vi "Scan from Function.vi"(0 "initial string":string, 1 "Syntax Format":T1, 11 "error in":errorcluster) -> (4 "resulting string":string, 6 "Variables Name":string[](array[string]), 8 "Variables Value":string[](array[string]), 15 "error out":errorcluster)   [LabVIEW 2019]
uses:
  Scan Syntax Format.ctl
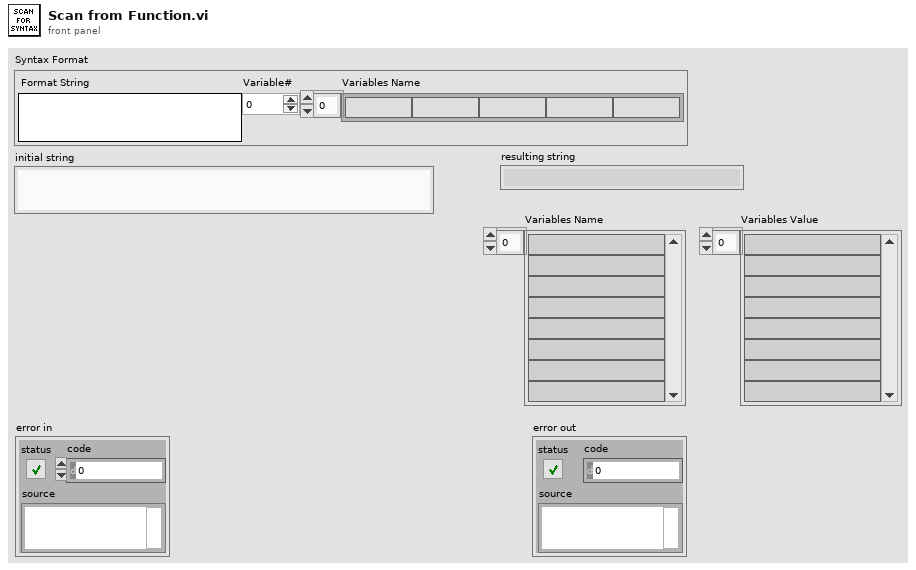
[diagram p1: front panel]
types:
  T1 = typedef "Scan Syntax Format.ctl" = cluster{"Format String":string, "Variable#":i32, "Variables Name":string[]}
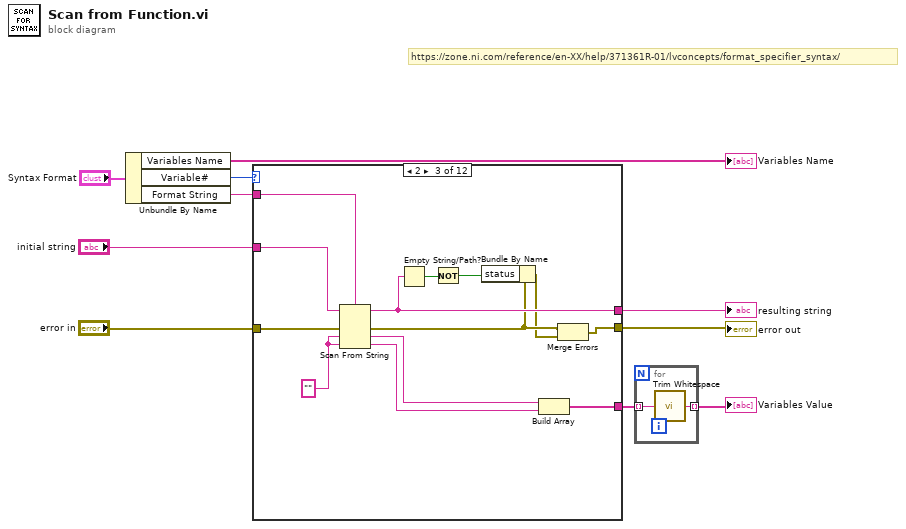
[diagram p0: block diagram]
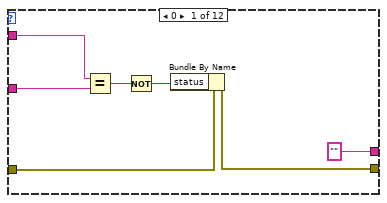
[diagram p2: hidden frame]
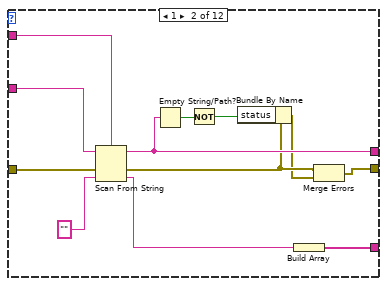
[diagram p3: hidden frame]
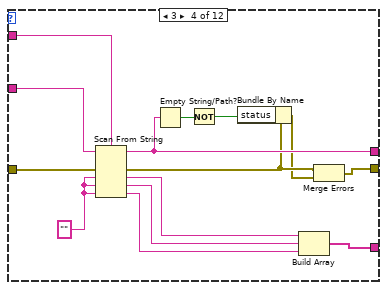
[diagram p4: hidden frame]
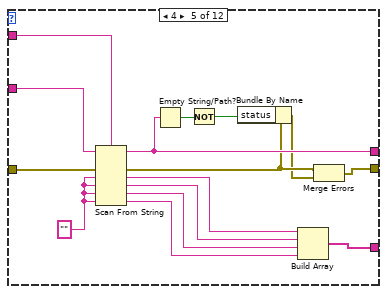
[diagram p5: hidden frame]
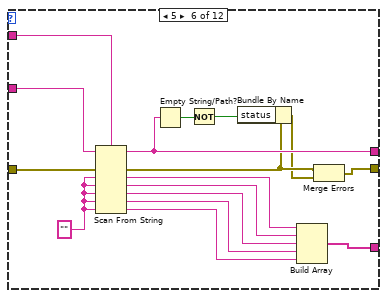
[diagram p6: hidden frame]
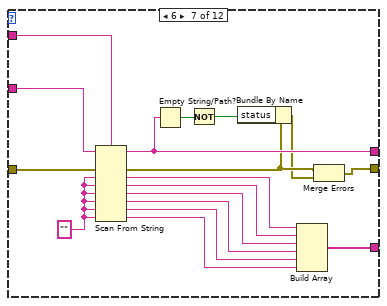
[diagram p7: hidden frame]
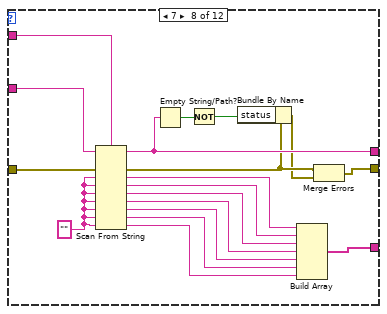
[diagram p8: hidden frame]
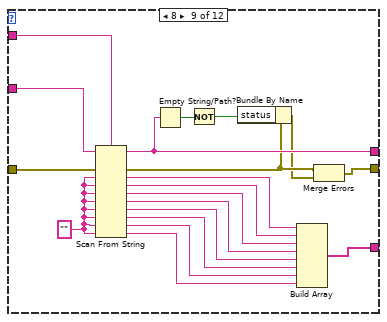
[diagram p9: hidden frame]
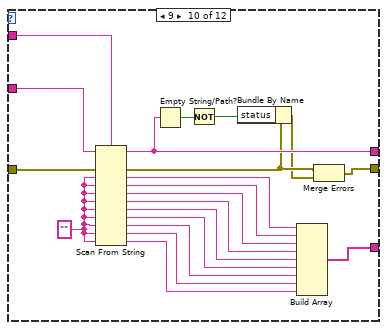
[diagram p10: hidden frame]
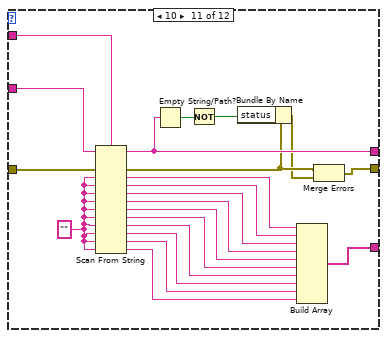
[diagram p11: hidden frame]
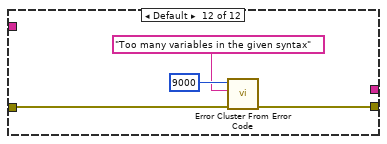
[diagram p12: hidden frame]
diagram:
  # "https://zone.ni.com/reference/en-XX/help/371361R-01/lvconcepts/format_specifier_syntax/"
  n1 = Unbundle By Name("Syntax Format") -> ("Variables Name"=→"Variables Name":string[], "Variable#"=w5:i32, "Format String"=w6:string)
  n2 = case shown="2" w5 {
    tunnel: "initial string" -> [w16 w29 w42 w56 w71 w87 w104 w122 w141 w161 w182 _]
    tunnel: "error in" -> [w14 w27 w41 w55 w70 w86 w103 w121 w140 w160 w181 w186]
    tunnel: ["" w26 w40 w54 w69 w85 w102 w120 w139 w159 w180 _] -> w8
    tunnel: [w13 w20 w34 w48 w63 w79 w96 w114 w133 w153 w174 w185] -> w1
    tunnel: w6 -> [w17 w23 w37 w51 w66 w82 w99 w117 w136 w156 w177 _]
    tunnel: [_ w18 w30 w43 w57 w72 w90 w108 w127 w147 w168 _] -> w3
    frame 0 {
      n3 = Equal?(x=w17, y=w16) -> (x = y?=w12:bool)
      n4 = Not(x=w12) -> (.not. x?=w11:bool)
      n5 = Bundle By Name(cluster=w14, "status"=w11) -> (w13:errorcluster)
    }
    frame 1 {
      n6 = Scan From String(format string=w23, input string=w29, error in=w27, default 1="") -> (remaining string=w26:string, error out=w22:errorcluster, output 1=w19:string)  [unwired: 1 in, 1 out]
      n7 = Empty String/Path?(string/path=w26) -> (empty?=w25:bool)
      n8 = Not(x=w25) -> (.not. x?=w24:bool)
      n9 = Bundle By Name(cluster=w22, "status"=w24) -> (w21:errorcluster)
      n10 = Build Array(w19) -> (w18:string[])
      n11 = Merge Errors(w22, w21) -> (w20:errorcluster)
    }
    frame 2 {
      w33 = ""
      n12 = Scan From String(format string=w37, input string=w42, error in=w41, default 1=w33, default 2=w33) -> (remaining string=w40:string, error out=w36:errorcluster, output 1=w32:string, output 2=w31:string)  [unwired: 1 in, 1 out]
      n13 = Empty String/Path?(string/path=w40) -> (empty?=w39:bool)
      n14 = Not(x=w39) -> (.not. x?=w38:bool)
      n15 = Bundle By Name(cluster=w36, "status"=w38) -> (w35:errorcluster)
      n16 = Build Array(w32, w31) -> (w30:string[])
      n17 = Merge Errors(w36, w35) -> (w34:errorcluster)
    }
    frame 3 {
      w47 = ""
      n18 = Scan From String(format string=w51, input string=w56, error in=w55, default 1=w47, default 2=w47, default 3=w47) -> (remaining string=w54:string, error out=w50:errorcluster, output 1=w46:string, output 2=w45:string, output 3=w44:string)  [unwired: 1 in, 1 out]
      n19 = Empty String/Path?(string/path=w54) -> (empty?=w53:bool)
      n20 = Not(x=w53) -> (.not. x?=w52:bool)
      n21 = Bundle By Name(cluster=w50, "status"=w52) -> (w49:errorcluster)
      n22 = Build Array(w46, w45, w44) -> (w43:string[])
      n23 = Merge Errors(w50, w49) -> (w48:errorcluster)
    }
    frame 4 {
      w62 = ""
      n24 = Scan From String(format string=w66, input string=w71, error in=w70, default 1=w62, default 2=w62, default 3=w62, default 4=w62) -> (remaining string=w69:string, error out=w65:errorcluster, output 1=w61:string, output 2=w60:string, output 3=w59:string, output 4=w58:string)  [unwired: 1 in, 1 out]
      n25 = Empty String/Path?(string/path=w69) -> (empty?=w68:bool)
      n26 = Not(x=w68) -> (.not. x?=w67:bool)
      n27 = Bundle By Name(cluster=w65, "status"=w67) -> (w64:errorcluster)
      n28 = Build Array(w61, w60, w59, w58) -> (w57:string[])
      n29 = Merge Errors(w65, w64) -> (w63:errorcluster)
    }
    frame 5 {
      w78 = ""
      n30 = Scan From String(format string=w82, input string=w87, error in=w86, default 1=w78, default 2=w78, default 3=w78, default 4=w78, default 5=w78) -> (remaining string=w85:string, error out=w81:errorcluster, output 1=w77:string, output 2=w76:string, output 3=w75:string, output 4=w74:string, output 5=w73:string)  [unwired: 1 in, 1 out]
      n31 = Empty String/Path?(string/path=w85) -> (empty?=w84:bool)
      n32 = Not(x=w84) -> (.not. x?=w83:bool)
      n33 = Bundle By Name(cluster=w81, "status"=w83) -> (w80:errorcluster)
      n34 = Build Array(w77, w76, w75, w74, w73) -> (w72:string[])
      n35 = Merge Errors(w81, w80) -> (w79:errorcluster)
    }
    frame 6 {
      w89 = ""
      n36 = Scan From String(format string=w99, input string=w104, error in=w103, default 1=w89, default 2=w89, default 3=w89, default 4=w89, default 5=w89, default 6=w89) -> (remaining string=w102:string, error out=w98:errorcluster, output 1=w95:string, output 2=w94:string, output 3=w93:string, output 4=w92:string, output 5=w91:string, output 6=w88:string)  [unwired: 1 in, 1 out]
      n37 = Empty String/Path?(string/path=w102) -> (empty?=w101:bool)
      n38 = Not(x=w101) -> (.not. x?=w100:bool)
      n39 = Bundle By Name(cluster=w98, "status"=w100) -> (w97:errorcluster)
      n40 = Build Array(w95, w94, w93, w92, w91, w88) -> (w90:string[])
      n41 = Merge Errors(w98, w97) -> (w96:errorcluster)
    }
    frame 7 {
      w105 = ""
      n42 = Scan From String(format string=w117, input string=w122, error in=w121, default 1=w105, default 2=w105, default 3=w105, default 4=w105, default 5=w105, default 6=w105, default 7=w105) -> (remaining string=w120:string, error out=w116:errorcluster, output 1=w113:string, output 2=w112:string, output 3=w111:string, output 4=w110:string, output 5=w109:string, output 6=w107:string, output 7=w106:string)  [unwired: 1 in, 1 out]
      n43 = Empty String/Path?(string/path=w120) -> (empty?=w119:bool)
      n44 = Not(x=w119) -> (.not. x?=w118:bool)
      n45 = Bundle By Name(cluster=w116, "status"=w118) -> (w115:errorcluster)
      n46 = Build Array(w113, w112, w111, w110, w109, w107, w106) -> (w108:string[])
      n47 = Merge Errors(w116, w115) -> (w114:errorcluster)
    }
    frame 8 {
      w123 = ""
      n48 = Scan From String(format string=w136, input string=w141, error in=w140, default 1=w123, default 2=w123, default 3=w123, default 4=w123, default 5=w123, default 6=w123, default 7=w123, default 8=w123) -> (remaining string=w139:string, error out=w135:errorcluster, output 1=w132:string, output 2=w131:string, output 3=w130:string, output 4=w129:string, output 5=w128:string, output 6=w126:string, output 7=w125:string, output 8=w124:string)  [unwired: 1 in, 1 out]
      n49 = Empty String/Path?(string/path=w139) -> (empty?=w138:bool)
      n50 = Not(x=w138) -> (.not. x?=w137:bool)
      n51 = Bundle By Name(cluster=w135, "status"=w137) -> (w134:errorcluster)
      n52 = Build Array(w132, w131, w130, w129, w128, w126, w125, w124) -> (w127:string[])
      n53 = Merge Errors(w135, w134) -> (w133:errorcluster)
    }
    frame 9 {
      w142 = ""
      n54 = Scan From String(format string=w156, input string=w161, error in=w160, default 1=w142, default 2=w142, default 3=w142, default 4=w142, default 5=w142, default 6=w142, default 7=w142, default 8=w142, default 9=w142) -> (remaining string=w159:string, error out=w155:errorcluster, output 1=w152:string, output 2=w151:string, output 3=w150:string, output 4=w149:string, output 5=w148:string, output 6=w146:string, output 7=w145:string, output 8=w144:string, output 9=w143:string)  [unwired: 1 in, 1 out]
      n55 = Empty String/Path?(string/path=w159) -> (empty?=w158:bool)
      n56 = Not(x=w158) -> (.not. x?=w157:bool)
      n57 = Bundle By Name(cluster=w155, "status"=w157) -> (w154:errorcluster)
      n58 = Build Array(w152, w151, w150, w149, w148, w146, w145, w144, w143) -> (w147:string[])
      n59 = Merge Errors(w155, w154) -> (w153:errorcluster)
    }
    frame 10 {
      w162 = ""
      n60 = Scan From String(format string=w177, input string=w182, error in=w181, default 1=w162, default 2=w162, default 3=w162, default 4=w162, default 5=w162, default 6=w162, default 7=w162, default 8=w162, default 9=w162, default 10=w162) -> (remaining string=w180:string, error out=w176:errorcluster, output 1=w173:string, output 2=w172:string, output 3=w171:string, output 4=w170:string, output 5=w169:string, output 6=w167:string, output 7=w166:string, output 8=w165:string, output 9=w164:string, output 10=w163:string)  [unwired: 1 in, 1 out]
      n61 = Empty String/Path?(string/path=w180) -> (empty?=w179:bool)
      n62 = Not(x=w179) -> (.not. x?=w178:bool)
      n63 = Bundle By Name(cluster=w176, "status"=w178) -> (w175:errorcluster)
      n64 = Build Array(w173, w172, w171, w170, w169, w167, w166, w165, w164, w163) -> (w168:string[])
      n65 = Merge Errors(w176, w175) -> (w174:errorcluster)
    }
    frame Default {
      n66 = call <vilib>:"Error Cluster From Error Code.vi"("error in (no error)"=w186, "error message (\"\")"="Too many variables in the given syntax" ("error message (\"\")"), "error code (0)"=9000) -> ("error out"=w185:errorcluster)  [unwired: 6 in]
    }
  }
  "resulting string" <- w8
  "error out" <- w1
  n67 = for {
    tunnel: w3 -> [w187] mode=indexing
    tunnel: [w188] -> w2 mode=indexing
    n68 = call <vilib>:"Trim Whitespace.vi"("string"=w187) -> ("trimmed string"=w188:string)  [unwired: 1 in]
  }
  "Variables Value" <- w2
